vi "DataLog Write String.vi"(0 "string":string, 5 "time (current)":dbl=nan format="%<%H:%M:%S%2u\n%Y/%m/%d>T", 7 "tag":string, 9 "tag index in (use tag)":i32=-1, 11 "error in (no error)":errorcluster) -> (10 "tag index out":i32, 15 "error out":errorcluster)   [LabVIEW 2012]
doc: "Writes a string value to a tag. The current time is used as timestamp if no custom time is wired. The current database must be live."
uses:
  typedefs/t_DataLog Live Tag Strings Methods.ctl
  typedefs/t_DataLog Tag Hash Methods.ctl
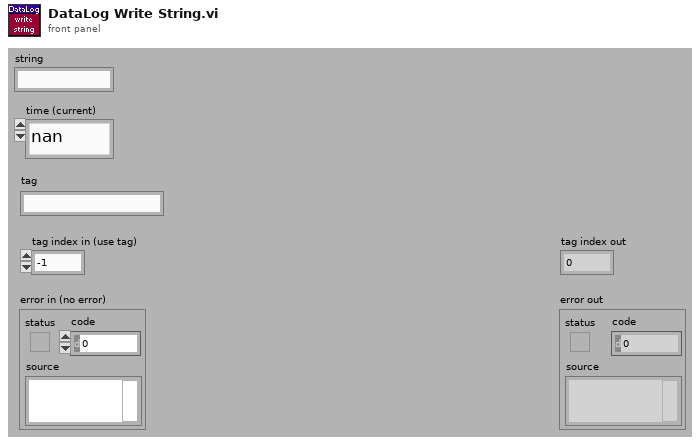
[diagram p1: front panel]
types:
  T1 = typedef "t_DataLog Live Tag Strings Methods.ctl" = enum16{"initialize", "rebuffer", "read", "write", "cleanup"}
  T2 = typedef "t_DataLog Tag Hash Methods.ctl" = enum16{"initialize", "add tag", "index tag", "lookup", "#tags", "cleanup", "write recovery", "read recovery", "delete recovery"}
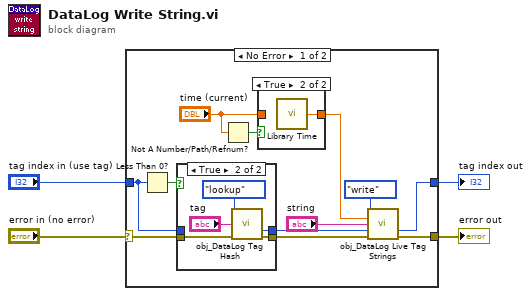
[diagram p0: block diagram]
diagram:
  n1 = case shown="No Error" "error in (no error)" {
    selector: "error in (no error)" -> [w11 w27]
    tunnel: [w8 w27] -> w3
    tunnel: "tag index in (use tag)" -> [w10 w26]
    tunnel: [w9 w26] -> w1
    frame No Error {
      n2 = Less Than 0?(x=w10) -> (x < 0?=w14:bool)
      n3 = case shown="True" w14 {
        tunnel: w11 -> [w20 w25]
        tunnel: [w20 w23] -> w13
        tunnel: [w19 w22] -> w12
        tunnel: w10 -> [w19 _]
        frame False {
        }
        frame True {
          n4 = call "obj_DataLog Tag Hash.vi"("method"=t_DataLog_Tag_Hash_Methods."lookup", "tag in"="tag", "error in (no error)"=w25) -> ("tag index out"=w22:i32, "error out"=w23:errorcluster)  [unwired: 9 in, 2 out]
        }
      }
      n5 = Not A Number/Path/Refnum?(number/path/refnum="time (current)") -> (NaN/Path/Refnum?=w7:bool)
      n6 = case shown="True" w7 {
        tunnel: "time (current)" -> [w17 _]
        tunnel: [w17 w18] -> w5
        frame False {
        }
        frame True {
          n7 = call "Library Time.vi"() -> ("time"=w18:dbl)  [unwired: 1 in]
        }
      }
      n8 = call "obj_DataLog Live Tag Strings.vi"("method"=t_DataLog_Live_Tag_Strings_Methods."write", "offset/time"=w5, "string in"="string", "tag index"=w12, "error in (no error)"=w13) -> ("dup tag index"=w9:i32, "error out"=w8:errorcluster)  [unwired: 7 in, 2 out]
    }
    frame Error {
    }
  }
  "error out" <- w3
  "tag index out" <- w1
